vi "limit change.vi"(1 "previous output":dbl, 2 "max change":dbl, 3 "value":dbl) -> (0 "output":dbl)   [LabVIEW 2009]
doc: "Ramps a value or array of values. In order for the array portion to function properly, it must be initialized (so that it knows how large the array is)"
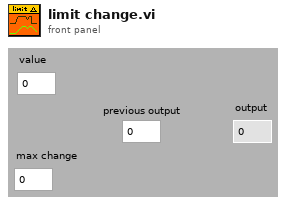
[diagram p1: front panel]
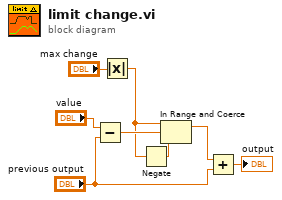
[diagram p0: block diagram]
diagram:
  n1 = Subtract(x="value", y="previous output") -> (x-y=w6:dbl)
  n2 = Absolute Value(x="max change") -> (abs(x)=w4:dbl)
  n3 = Negate(x=w4) -> (-x=w8:dbl)
  n4 = In Range and Coerce(upper limit=w4, x=w6, lower limit=w8) -> (coerced(x)=w3:dbl)  [unwired: 1 out]
  n5 = Add(x=w3, y="previous output") -> (x+y=→"output":dbl)
